vi "Rectangle Contains Point.vi"(4 "Point":cluster{"x":dbl, "y":dbl}, 5 "Rectangle":T1) -> (1 "Contained?":bool)   [LabVIEW 2015]
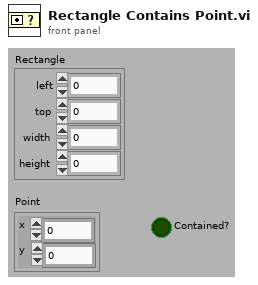
[diagram p1: front panel]
types:
  T1 = cluster{"left":dbl, "top":dbl, "width":dbl, "height":dbl}
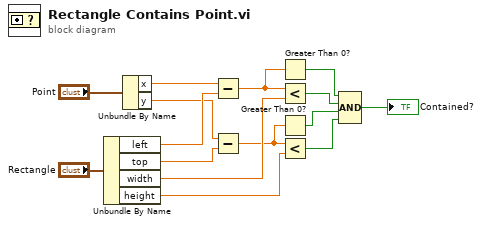
[diagram p0: block diagram]
diagram:
  n1 = Unbundle By Name("Rectangle") -> ("left"=w12:dbl, "top"=w10:dbl, "width"=w9:dbl, "height"=w8:dbl)
  n2 = Unbundle By Name("Point") -> ("x"=w13:dbl, "y"=w11:dbl)
  n3 = Subtract(x=w13, y=w12) -> (x-y=w7:dbl)
  n4 = Subtract(x=w11, y=w10) -> (x-y=w6:dbl)
  n5 = Greater Than 0?(x=w7) -> (x > 0?=w5:bool)
  n6 = Less?(x=w7, y=w9) -> (x < y?=w4:bool)
  n7 = Greater Than 0?(x=w6) -> (x > 0?=w3:bool)
  n8 = Less?(x=w6, y=w8) -> (x < y?=w2:bool)
  n9 = Compound Arithmetic op=AND(w5, w4, w3, w2) -> (→"Contained?":bool)
